vi "Arrange VIWin - Space FP Controls.vi"(0 "controls":refnum<vi>[](array[refnum]), 1 "FP objects arrangement info":T1, 5 "left bound":i32, 7 "max vertical rectangle delta for controls from the top row":i16, 11 "error in":errorcluster) -> (4 "Max right location":i32, 15 "error out":errorcluster)   [LabVIEW 2012, in "Arrange VI Window.lvlib"]
uses:
  Arrange VI Window.lvlib
  Arrange VIWin - FP Objects Arrangement Info.ctl
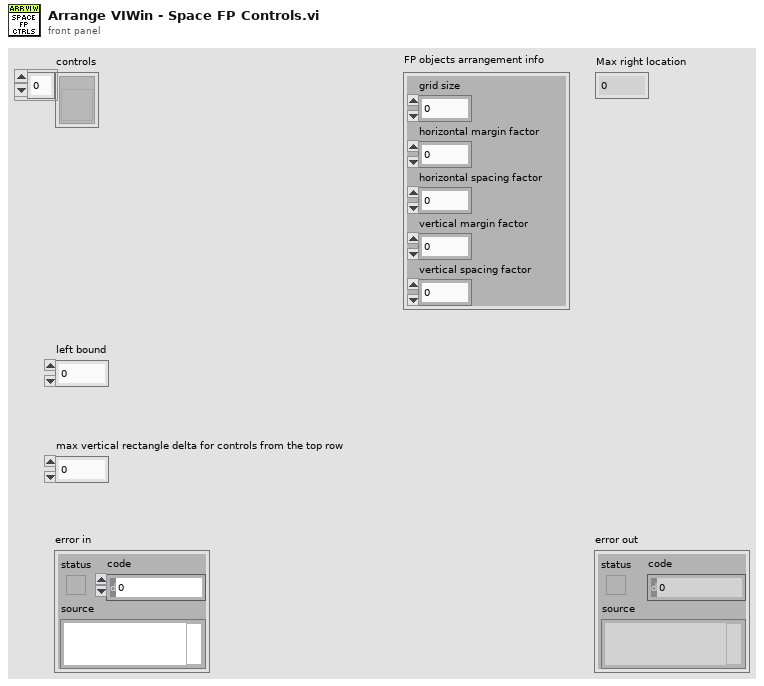
[diagram p1: front panel]
types:
  T1 = typedef "Arrange VI Window.lvlib/Arrange VIWin - FP Objects Arrangement Info.ctl" = cluster{"grid size":i32, "horizontal margin factor":i32, "horizontal spacing factor":i32, "vertical margin factor":i32, "vertical spacing factor":i32}
  T2 = typedef "LVRectTypeDef.ctl" = cluster{"Left":i16, "Top":i16, "Right":i16, "Bottom":i16}
  T3 = cluster{"Left":i32, "Top":i32, "Right":i32, "Bottom":i32}
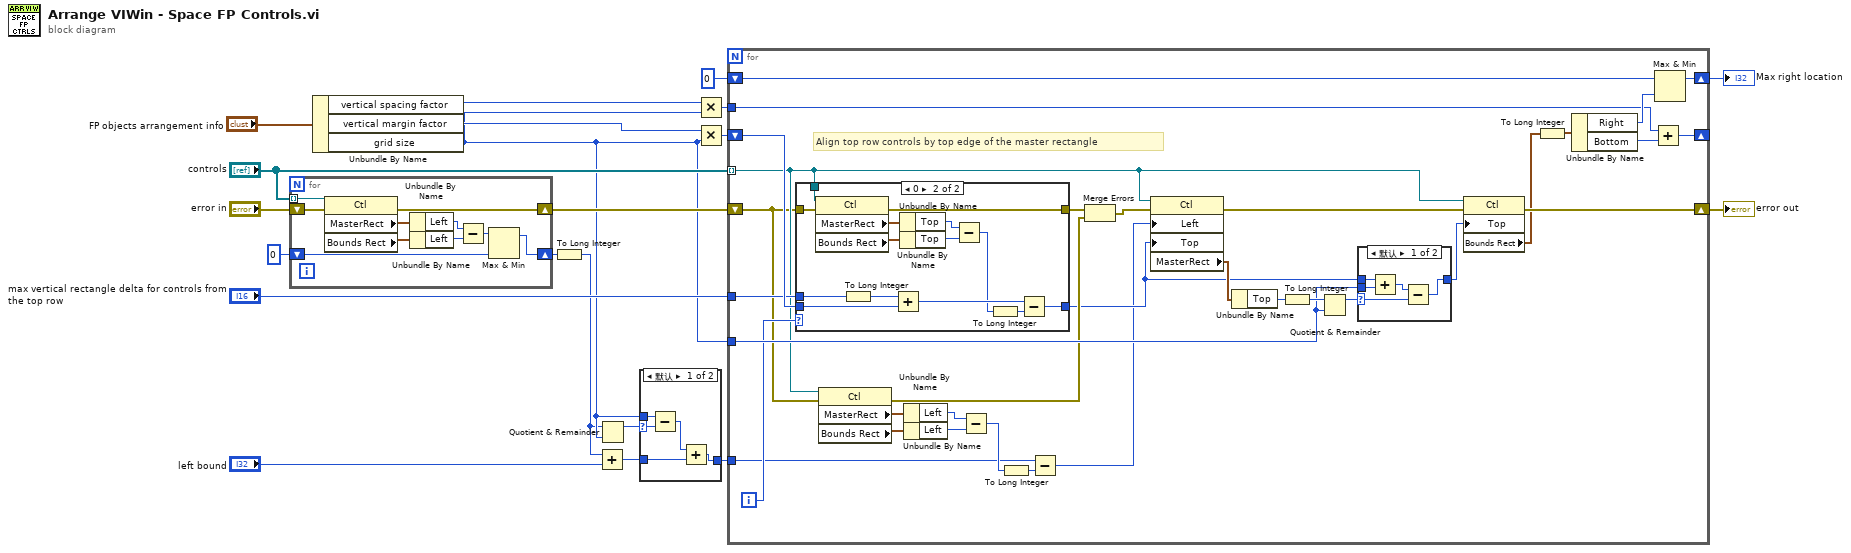
[diagram p0: block diagram]
diagram:
  n1 = for {
    shift-right: [w27] -> w12
    shift-left: "error in" -> [w28]
    shift-right: [w23] -> w9
    shift-left: i16 0 -> [w22]
    tunnel: "controls" -> [w21] mode=indexing
    n2 = property class="Ctl"(reference=w21, error in=w28) -> (error out=w27:errorcluster, "MasterRect"=w30:T2, "Bounds Rect"=w29:T2)  [unwired: 1 out]
    n3 = Unbundle By Name(w30) -> ("Left"=w25:i16)
    n4 = Unbundle By Name(w29) -> ("Left"=w26:i16)
    n5 = Subtract(x=w25, y=w26) -> (x-y=w24:i16)
    n6 = Max & Min(x=w24, y=w22) -> (max(x,y)=w23:i16)  [unwired: 1 out]
  }
  n7 = Unbundle By Name("FP objects arrangement info") -> ("vertical spacing factor"=w17:i32, "vertical margin factor"=w16:i32, "grid size"=w7:i32)
  n8 = To Long Integer(number=w9) -> (32bit integer=w4:i32)
  n9 = Add(x=w4, y="left bound") -> (x+y=w6:i32)
  n10 = Quotient & Remainder(x=w4, y=w7) -> (x-y*floor(x/y)=w8:i32)  [unwired: 1 out]
  n11 = case shown="默认" w8 {
    selector: w8 -> [w35 _]
    tunnel: w7 -> [w34 _]
    tunnel: [w33 w36] -> w3
    tunnel: w6 -> [w31 w36]
    frame Default {
      n12 = Subtract(x=w34, y=w35) -> (x-y=w32:i32)
      n13 = Add(x=w32, y=w31) -> (x+y=w33:i32)
    }
    frame 0 {
    }
  }
  n14 = Multiply(x=w17, y=w7) -> (x*y=w15:i32)
  n15 = Multiply(x=w16, y=w7) -> (x*y=w14:i32)
  n16 = for {
    tunnel: "controls" -> [w45] mode=indexing
    shift-right: [w69] -> _
    shift-left: w14 -> [w51]
    shift-right: [w59] -> w20
    shift-left: w12 -> [w44]
    shift-right: [w68] -> w19
    shift-left: 0 -> [w67]
    tunnel: w7 -> [w53]
    tunnel: w15 -> [w64]
    tunnel: "max vertical rectangle delta for controls from the top row" -> [w50]
    tunnel: w3 -> [w40]
    i -> [w52]
    # "Align top row controls by top edge of the master rectangle"
    n17 = case shown="0" w52 {
      tunnel: w44 -> [w71 w85]
      tunnel: [w71 w84] -> w54
      tunnel: w45 -> [_ w83]
      tunnel: [w70 w72] -> w41
      tunnel: w51 -> [w70 w73]
      tunnel: w50 -> [_ w78]
      frame Default {
      }
      frame 0 {
        n18 = property class="Ctl"(reference=w83, error in=w85) -> (error out=w84:errorcluster, "MasterRect"=w82:T2, "Bounds Rect"=w81:T2)  [unwired: 1 out]
        n19 = To Long Integer(number=w78) -> (32bit integer=w77:i32)
        n20 = Add(x=w77, y=w73) -> (x+y=w76:i32)
        n21 = Unbundle By Name(w82) -> ("Top"=w79:i16)
        n22 = Unbundle By Name(w81) -> ("Top"=w80:i16)
        n23 = Subtract(x=w79, y=w80) -> (x-y=w75:i16)
        n24 = To Long Integer(number=w75) -> (32bit integer=w74:i32)
        n25 = Subtract(x=w76, y=w74) -> (x-y=w72:i32)
      }
    }
    n26 = property class="Ctl"(reference=w45, error in=w44) -> (error out=w42:errorcluster, "MasterRect"=w49:T2, "Bounds Rect"=w48:T2)  [unwired: 1 out]
    n27 = Unbundle By Name(w49) -> ("Left"=w39:i16)
    n28 = Unbundle By Name(w48) -> ("Left"=w38:i16)
    n29 = Subtract(x=w39, y=w38) -> (x-y=w47:i16)
    n30 = To Long Integer(number=w47) -> (32bit integer=w46:i32)
    n31 = Subtract(x=w40, y=w46) -> (x-y=w37:i32)
    n32 = Merge Errors(w54, w42) -> (w43:errorcluster)
    n33 = property class="Ctl"(reference=w45, error in=w43, "Left"=w37, "Top"=w41) -> (error out=w60:errorcluster, "MasterRect"=w62:T2)  [unwired: 1 out]
    n34 = Unbundle By Name(w62) -> ("Top"=w61:i16)
    n35 = To Long Integer(number=w61) -> (32bit integer=w57:i32)
    n36 = Quotient & Remainder(x=w57, y=w53) -> (x-y*floor(x/y)=w55:i32)  [unwired: 1 out]
    n37 = case shown="默认" w55 {
      selector: w55 -> [w87 _]
      tunnel: [w86 w91] -> w56
      tunnel: w41 -> [w90 w91]
      tunnel: w53 -> [w89 _]
      frame Default {
        n38 = Add(x=w90, y=w89) -> (x+y=w88:i32)
        n39 = Subtract(x=w88, y=w87) -> (x-y=w86:i32)
      }
      frame 0 {
      }
    }
    n40 = property class="Ctl"(reference=w45, error in=w60, "Top"=w56) -> (error out=w59:errorcluster, "Bounds Rect"=w58:T2)  [unwired: 1 out]
    n41 = To Long Integer(number=w58) -> (32bit integer=w63:T3)
    n42 = Unbundle By Name(w63) -> ("Right"=w66:i32, "Bottom"=w65:i32)
    n43 = Add(x=w64, y=w65) -> (x+y=w69:i32)
    n44 = Max & Min(x=w67, y=w66) -> (max(x,y)=w68:i32)  [unwired: 1 out]
  }
  "Max right location" <- w19
  "error out" <- w20
